vi "PostCopyScripting.vi"(10 "MetaDataObj":refnum<class "MetaDataObj.lvclass">, 11 "User Project":refnum<vi>) -> ()   [LabVIEW 2013, in "FixedChannelTBModuleDecideFeatures.lvclass"]
uses:
  FixedChannelTBModuleDecideFeatures.lvclass
  <resource>/dialog/NewProjectWizard/MetaDataObj/MetaDataObj.lvclass
  FixedChannelTBModuleDecideFeatures.lvclass/FixedChannelTBModuleDecideFeatures.ctl
  Read component name.vi
  Read Channel Specification.vi
  <vilib>/NI/Tag Bus Data Framework/control module/script/control module data interface generator.lvlib
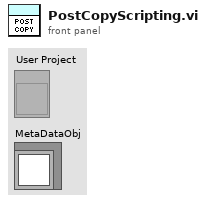
[diagram p1: front panel]
types:
  T1 = typedef "channel configuration.ctl" = cluster{"Name":string, "channel classification":T2, "data type":T3}
  T2 = typedef "TBM channel.lvclass/channel classification.ctl" = enum16{"input data", "output data", "processing parameter", "processing result"}
  T3 = typedef "tag bus.lvlib/tag descriptor.lvclass/Data Type.ctl" = enum16{"Double", "Single", "I64", "I32", "I16", "I8", "U64", "U32", "U16", "U8", "Boolean", "String", "Array of Double", "Array of Single", "Array of I64", "Array of I32", "Array of I16", "Array of I8", "Array of U64", "Array of U32", "Array of U16", "Array of U8", "Array of Boolean", "Array of String"}
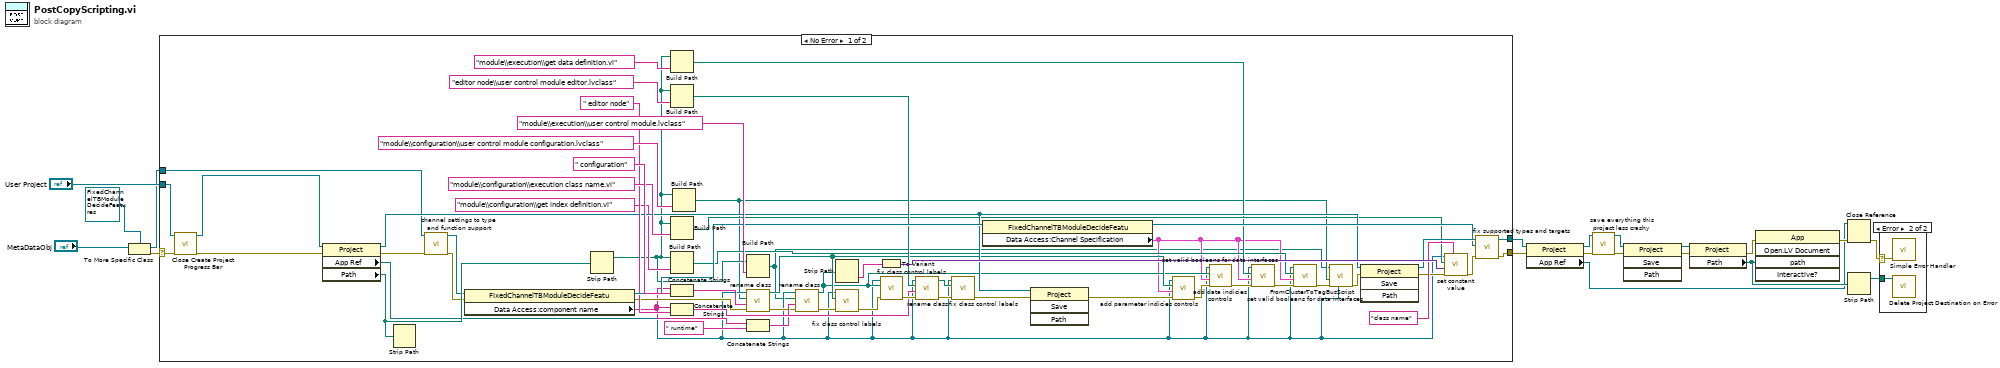
[diagram p0: block diagram]
diagram:
  n1 = To More Specific Class(target class=refnum<class "FixedChannelTBModuleDecideFeatures.lvclass"> refnum ("DecideProjectFeatures.lvclass"), reference="MetaDataObj") -> (specific class reference=w10:refnum<class "FixedChannelTBModuleDecideFeatures.lvclass">, error out=w17:errorcluster)  [unwired: 1 in]
  n2 = case shown="No Error" w17 {
    selector: w17 -> [w35 w78]
    tunnel: [w58 w79] -> w2
    tunnel: "User Project" -> [w36 w79]
    tunnel: [w59 w78] -> w3
    tunnel: w10 -> [w44 _]
    frame No Error {
      n3 = call <resource>:"Close Create Project Progress Bar.vi"("error in (no error)"=w35, "Project"=w36) -> ("error out"=w34:errorcluster, "dup Project"=w33:refnum<vi>)  [unwired: 8 in]
      n4 = property class="Project"(reference=w33, error in=w34) -> (reference out=w49:refnum<vi>, error out=w43:errorcluster, "App Ref"=w22:refnum<vi>, "Path"=w48:path)
      n5 = Strip Path(path=w48) -> ()  [unwired: 2 out]
      n6 = call "channel settings to type and function support.vi"("error in"=w43, "FixedChannelTBModuleDecideFeatures in"=w44) -> ("error out"=w46:errorcluster, "FixedChannelTBModuleDecideFeatures out"=w45:refnum<class "FixedChannelTBModuleDecideFeatures.lvclass">)  [unwired: 8 in]
      n7 = property class="FixedChannelTBModuleDecideFeatu"(reference=w45, error in=w46) -> (reference out=w74:refnum<class "FixedChannelTBModuleDecideFeatures.lvclass">, error out=w47:errorcluster, "Data Access:component name"=w38:string)
      n8 = Strip Path(path=w48) -> (stripped path=w30:path)  [unwired: 1 out]
      n9 = Build Path(base path=w30, name or relative path="module\\execution\\get data definition.vi") -> (appended path=w28:path)
      n10 = Build Path(base path=w30, name or relative path="editor node\\user control module editor.lvclass") -> (appended path=w65:path)
      n11 = Build Path(base path=w30, name or relative path="module\\configuration\\execution class name.vi") -> (appended path=w42:path)
      n12 = Build Path(base path=w30, name or relative path="module\\configuration\\get index definition.vi") -> (appended path=w26:path)
      n13 = Concatenate Strings(w38, " configuration" ("string")) -> (w56:string)
      n14 = Concatenate Strings(w38, " editor node" ("string")) -> (w60:string)
      n15 = Build Path(base path=w30, name or relative path="module\\configuration\\user control module configuration.lvclass") -> (appended path=w21:path)
      n16 = Build Path(base path=w30, name or relative path="module\\execution\\user control module.lvclass") -> (appended path=w20:path)
      n17 = call "rename class.vi"("error in"=w47, "new name"=w56, "class path"=w21, "Application in"=w22) -> ("error out"=w52:errorcluster, "New Library Path"=w41:path)  [unwired: 6 in]
      n18 = Concatenate Strings(w38, " runtime" ("string")) -> (w53:string)
      n19 = call "rename class.vi"("error in"=w52, "new name"=w53, "class path"=w20, "Application in"=w22) -> ("error out"=w68:errorcluster, "New Library Path"=w39:path)  [unwired: 6 in]
      n20 = Strip Path(path=w39) -> (name=w55:string)  [unwired: 1 out]
      n21 = call "fix class control labels.vi"("error in"=w68, "class to load"=w41, "Application in"=w22) -> ("error out"=w67:errorcluster)  [unwired: 8 in]
      n22 = To Variant(anything=w55) -> (Variant=w73:variant)
      n23 = call "fix class control labels.vi"("error in"=w67, "class to load"=w39, "Application in"=w22) -> ("error out"=w62:errorcluster)  [unwired: 8 in]
      n24 = call "rename class.vi"("error in"=w62, "new name"=w60, "class path"=w65, "Application in"=w22) -> ("error out"=w63:errorcluster, "New Library Path"=w64:path)  [unwired: 6 in]
      n25 = call "fix class control labels.vi"("error in"=w63, "class to load"=w64, "Application in"=w22) -> ("error out"=w37:errorcluster)  [unwired: 8 in]
      n26 = property class="FixedChannelTBModuleDecideFeatu"(reference=w74) -> (reference out=w51:refnum<class "FixedChannelTBModuleDecideFeatures.lvclass">, "Data Access:Channel Specification"=w25:T1[])  [unwired: 1 in, 1 out]
      n27 = invoke class="Project" method="Save"(reference=w49, error in=w37) -> (error out=w50:errorcluster)  [unwired: 2 in, 3 out]
      n28 = call "add parameter indicies controls.vi"("error in"=w50, "Channels to create"=w25, "cfg class path"=w41, "Application in"=w22) -> ("error out"=w40:errorcluster)  [unwired: 7 in]
      n29 = call "add data indicies controls.vi"("error in"=w40, "Channels to create"=w25, "runtime class path"=w39, "Application in"=w22) -> ("error out"=w29:errorcluster)  [unwired: 7 in]
      n30 = call "set valid booleans for data interfaces.vi"("error in"=w29, "Channel Specification"=w25, "vi path"=w28, "Application in"=w22) -> ("error out"=w27:errorcluster)  [unwired: 7 in]
      n31 = call "set valid booleans for data interfaces.vi"("error in"=w27, "Channel Specification"=w25, "vi path"=w26, "Application in"=w22) -> ("error out"=w24:errorcluster)  [unwired: 7 in]
      n32 = call <vilib>:"FromClusterToTagBusScript.vi"("application reference (local)"=w22, "error in"=w24, "configuration class path"=w21, "runtime class path"=w20) -> ("error out"=w23:errorcluster)  [unwired: 7 in]
      n33 = invoke class="Project" method="Save"(reference=w49, error in=w23) -> (reference out=w69:refnum<vi>, error out=w70:errorcluster)  [unwired: 2 in, 2 out]
      n34 = call "set constant value.vi"("control name"="class name", "error in"=w70, "data to set"=w73, "vi path"=w42, "Application in"=w22) -> ("error out"=w57:errorcluster)  [unwired: 6 in]
      n35 = call "fix supported types and targets.vi"("error in"=w57, "DecideProjectFeatures in"=w51, "User Project in"=w69) -> ("error out"=w59:errorcluster, "User Project out"=w58:refnum<vi>)  [unwired: 7 in]
    }
    frame Error {
    }
  }
  n36 = property class="Project"(reference=w2, error in=w3) -> (reference out=w7:refnum<vi>, error out=w8:errorcluster, "App Ref"=w1:refnum<vi>)
  n37 = call "save everything this project less crashy.vi"("error in"=w8, "Project in"=w7) -> ("error out"=w4:errorcluster, "Project out"=w9:refnum<vi>)  [unwired: 8 in]
  n38 = invoke class="Project" method="Save"(reference=w9, error in=w4) -> (reference out=w13:refnum<vi>, error out=w14:errorcluster)  [unwired: 2 in, 2 out]
  n39 = property class="Project"(reference=w13, error in=w14) -> (error out=w16:errorcluster, "Path"=w11:path)  [unwired: 1 out]
  n40 = invoke class="App" method="Open.LV Document"(error in=w16, "path"=w11) -> (error out=w15:errorcluster)  [unwired: 3 in, 4 out]
  n41 = Close Reference(reference=w1, error in (no error)=w15) -> (error out=w6:errorcluster)
  n42 = Strip Path(path=w11) -> (stripped path=w5:path)  [unwired: 1 out]
  n43 = case shown="Error" w6 {
    selector: w6 -> [_ w80]
    tunnel: w5 -> [_ w81]
    frame No Error {
    }
    frame Error {
      n44 = call <vilib>:"Simple Error Handler.vi"("error in (no error)"=w80) -> ()  [unwired: 4 in, 5 out]
      n45 = call <resource>:"Delete Project Destination on Error.vi"("Project Destination Root"=w81) -> ()  [unwired: 11 in]
    }
  }
